vi "start condition (SubVI).vi"   [LabVIEW 2019]
uses:
  <vilib>/rvi/eio/common/nirviEmuTemplateMethod_errors.vi
  <vilib>/eio/EIONode/EIONode.xnode
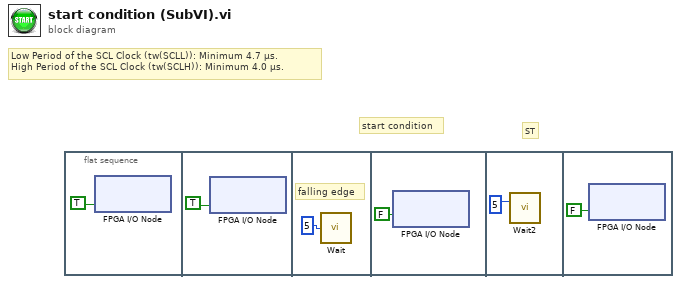
[diagram p0: block diagram]
diagram:
  # "Low Period of the SCL Clock (tw(SCLL)): Minimum 4.7 µs.\nHigh Period of the SCL Clock (tw(SCLH)): Minimum 4.0 µs."
  # "ST"
  # "start condition"
  n1 = flat-sequence {
    frame #0 {
      n2 = xnode "FPGA I/O Node"("SDA"=TRUE) -> ()  [unwired: 1 in, 1 out]
    }
    frame #1 {
      n3 = xnode "FPGA I/O Node"("SCL"=TRUE) -> ()  [unwired: 1 in, 1 out]
    }
    frame #2 {
      # "falling edge"
      n4 = call "Wait"("Count(uSec)"=u32 5 ("Count(Ticks)")) -> ()  [unwired: 1 out]
    }
    frame #3 {
      n5 = xnode "FPGA I/O Node"("SDA"=FALSE) -> ()  [unwired: 1 in, 1 out]
    }
    frame #4 {
      n6 = call "Wait2"("Count(uSec)"=u32 5 ("Count(Ticks)")) -> ()  [unwired: 1 out]
    }
    frame #5 {
      n7 = xnode "FPGA I/O Node"("SCL"=FALSE) -> ()  [unwired: 1 in, 1 out]
    }
  }
